vi "Пример осциллограммы.vi"() -> ()   [LabVIEW 2017]
doc: "This VI is used in Exercise 9-6 of the LabVIEW Basics I Course.\n\nYou choose an ASCII or binary waveform string. Then the string control shows the appropriate waveform data. Then the VI converts that string to an array of numbers and plots those values in a graph."
panel:
  out "кол-во байт в строке":i32
  in  "Источник данных":bool
  in  "Формат данных":bool
  out "График осцилограммы данных":dbl[](graph)
  out "Строка осциллограммы данных":string
  in  "Binary String":string="#3128·улЪФЪвевЮЭЯабаЯЯЯаааЯЯЯаH\f\u0014%+%\u001d\u001a\u001d!\" \u001f\u001e\u001f   \u001f\u001f\u001f   \u001f·улЪФЪвевЮЭЯабаЯЯЯаааЯЯЯаH\f\u0014%+%\u001d\u001a\u001d!\" \u001f\u001e\u001f   \u001f\u001f\u001f   \u001f·улЪФЪвевЮЭЯабаЯЯЯаааЯЯЯаH\f\u0014\n"
  in  "ASCII String":string="CURVE 4.3748,0.9054E1,0.8429E1,7.1068,6.6331,7.0970,7.7300,7.9161,7.6677,7.3702,7.3012,7.4318,7.5704,7.5936,7.5261,7.4620,7.4556,7.4901,7.5197,7.5203,7.5026,7.4892,7.4901,7.4993,7.5051,-4.3754,-0.9055E1,-0.8429E1,-7.1071,-6.6335,-7.0970,-7.7303,-7.9165,-7.6680,-7.3705,-7.3015,-7.4318,-7.5707,-7.5939,-7.5264,-7.4623,-7.4559,-7.4904,-7.5197,-7.5206,-7.5029,-7.4895,-7.4904,-7.4993,-7.5051,4.3748,0.9054E1,0.8429E1,7.1068,6.6331,7.0970,7.7300,7.9161,7.6677,7.3702,7.3012,7.4318,7.5704,7.5936,7.5261,7.4620,7.4556,7.4901,7.5197,7.5203,7.5026,7.4892,7.4901,7.4993,7.5051,-4.3754,-0.9055E1,-0.8429E1,-7.1071,-6.6335,-7.0970,-7.7303,-7.9165,-7.6680,-7.3705,-7.3015,-7.4318,-7.5707,-7.5939,-7.5264,-7.4623,-7.4559,-7.4904,-7.5197,-7.5206,-7.5029,-7.4895,-7.4904,-7.4993,-7.5051,4.3748,0.9054E1,0.8429E1,7.1068,6.6331,7.0970,7.7300,7.9161,7.6677,7.3702,7.3012,7.4318,7.5704,7.5936,7.5261,7.4620,7.4556,7.4901,7.5197,7.5203,7.5026,7.4892,7.4901,7.4993,7.5051,-4.3754,-0.9055E1,-0.8429E1\n"
  # "Двоичный"
  # "Имитатор"
  # "ASCII"
  # "GPIB"
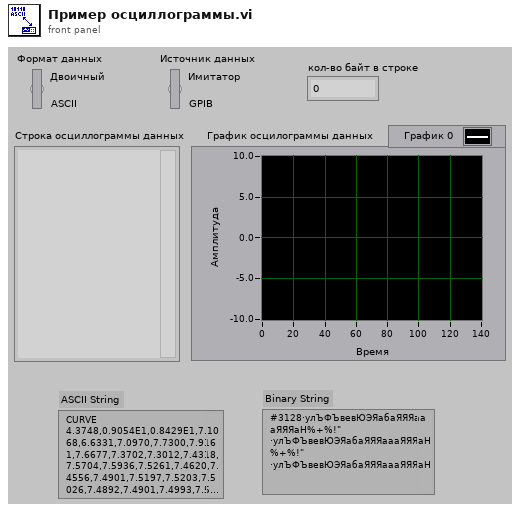
[diagram p1: front panel]
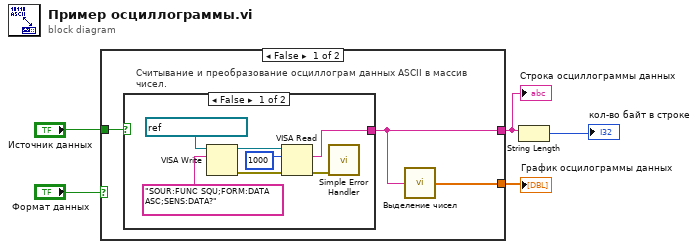
[diagram p0: block diagram]
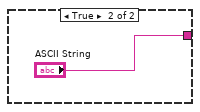
[diagram p2: hidden frame]
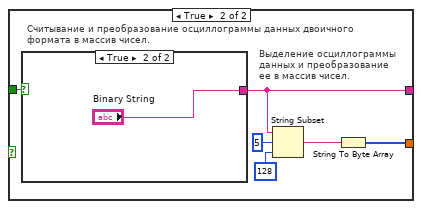
[diagram p3: hidden frame]
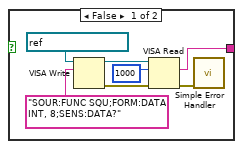
[diagram p4: hidden frame]
diagram:
  n1 = case shown="False" "Формат данных" {
    tunnel: [w7 w18] -> w3
    tunnel: [w8 w17] -> w1
    tunnel: "Источник данных" -> [w6 w19]
    frame False {
      # "Считывание и преобразование осциллограм данных ASCII в массив чисел."
      n2 = case shown="False" w6 {
        tunnel: [w11 "ASCII String"] -> w7
        frame False {
          n3 = VISA Write(VISA resource name=refnum<visa-resource-name> "GPIB::2::INSTR", write buffer="SOUR:FUNC SQU;FORM:DATA ASC;SENS:DATA?") -> (VISA resource name out=w14:refnum<visa-resource-name>, error out=w15:errorcluster)  [unwired: 1 in, 1 out]
          n4 = VISA Read(VISA resource name=w14, byte count=u32 1000 ("byte count (0)"), error in (no error)=w15) -> (read buffer=w11:string, error out=w12:errorcluster)  [unwired: 2 out]
          n5 = call <vilib>:"Simple Error Handler.vi"("error in (no error)"=w12) -> ()  [unwired: 4 in, 5 out]
        }
        frame True {
        }
      }
      n6 = call "Выделение чисел.vi"("Строка"=w7) -> ("Массив данных двойной точности"=w8:dbl[])
    }
    frame True {
      # "Выделение осциллограммы данных и преобразование ее в массив чисел."
      # "Считывание и преобразование осциллограммы данных двоичного формата в массив чисел."
      n7 = case shown="True" w19 {
        tunnel: [w26 "Binary String"] -> w18
        frame False {
          n8 = VISA Write(VISA resource name=refnum<visa-resource-name> "GPIB::2::INSTR", write buffer="SOUR:FUNC SQU;FORM:DATA INT, 8;SENS:DATA?") -> (VISA resource name out=w27:refnum<visa-resource-name>, error out=w28:errorcluster)  [unwired: 1 in, 1 out]
          n9 = VISA Read(VISA resource name=w27, byte count=u32 1000 ("byte count (0)"), error in (no error)=w28) -> (read buffer=w26:string, error out=w29:errorcluster)  [unwired: 2 out]
          n10 = call <vilib>:"Simple Error Handler.vi"("error in (no error)"=w29) -> ()  [unwired: 4 in, 5 out]
        }
        frame True {
        }
      }
      n11 = String Subset(string=w18, offset (0)=5, length (rest)=128) -> (substring=w22:string)
      n12 = String To Byte Array(string=w22) -> (unsigned byte array=w17:u8[])
    }
  }
  "Строка осциллограммы данных" <- w3
  "График осцилограммы данных" <- w1
  n13 = String Length(string=w3) -> (length=→"кол-во байт в строке":i32)
